vi "Create BufferedArray.vi"(8 "error in (no error)":errorcluster, 9 "Maximum Buffer Increment (65536)":i32=65536, 10 "Minimum Buffer Size (256)":i32=256) -> (0 "error out":errorcluster, 3 "BufferedArray out":refnum<class "BufferedArray.lvclass">)   [LabVIEW 2017, in "LapDog.Collections.v0.Lists.Implementations.lvlib" / "BufferedArray.lvclass"]
uses:
  BufferedArray.lvclass
  BufferedArray.lvclass/BufferedArray.ctl
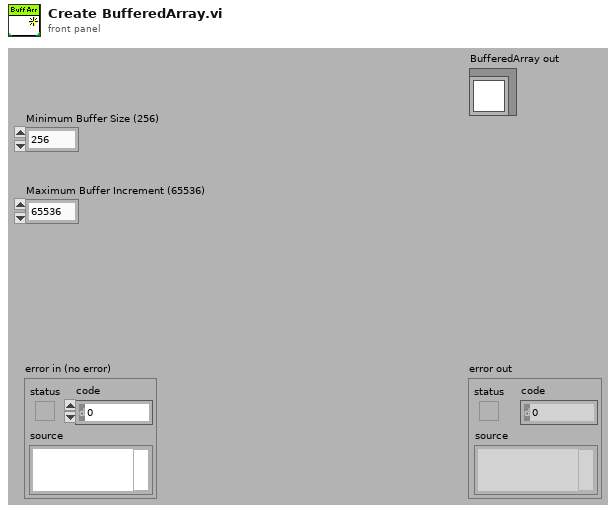
[diagram p1: front panel]
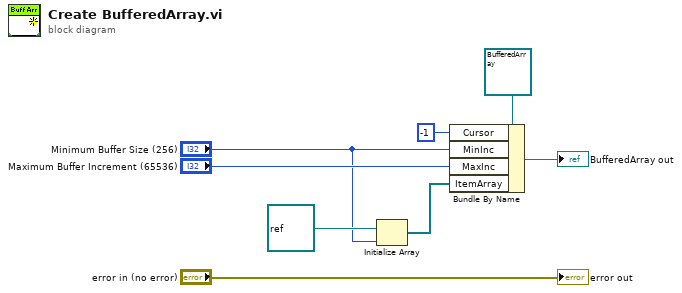
[diagram p0: block diagram]
diagram:
  n1 = Initialize Array(refnum<class> refnum ("LabVIEW Object"), "Minimum Buffer Size (256)") -> (w2:refnum<class>[])
  n2 = Bundle By Name(cluster=refnum<class "BufferedArray.lvclass"> refnum ("BufferedArray in"), "Cursor"=-1 ("Count"), "MinInc"="Minimum Buffer Size (256)", "MaxInc"="Maximum Buffer Increment (65536)", "ItemArray"=w2) -> (→"BufferedArray out":refnum<class "BufferedArray.lvclass">)
  "error out" <- "error in (no error)"
